vi "sqlite3_errmsg.vi"(8 "error in (no error)":errorcluster, 11 "psqlite":i64) -> (0 "error out":errorcluster, 3 "return type":string)   [LabVIEW 2014, in "SQLite3LV.lvlib"]
uses:
  SQLite3LV.lvlib
  sqlite3_64.dll
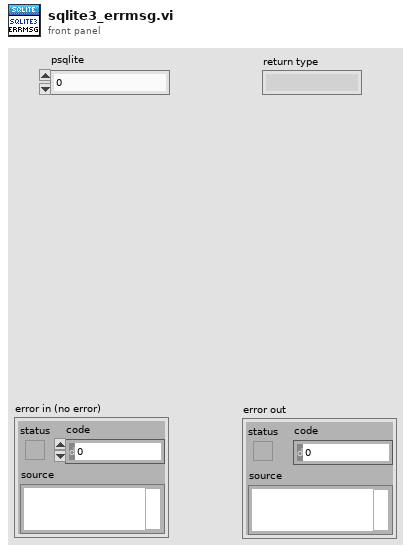
[diagram p1: front panel]
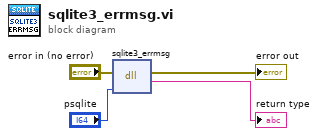
[diagram p0: block diagram]
diagram:
  n1 = dll-call lib="C:/Users/BobUser/Desktop/LVTables/sqlite3**.*" fn="sqlite3_errmsg"(error in="error in (no error)", "psqlite"="psqlite") -> (error out=→"error out":errorcluster, "return type"=→"return type":string)  [unwired: 3 in, 1 out]
